vi "SetParameter.vi"(7 "Camera Parameter":T1, 8 "error in (no error)":errorcluster, 10 "Value":i32, 11 "Stream in":refnum<class "Stream.lvclass">) -> (0 "error out":errorcluster, 1 "Set Value":i32, 3 "Stream (Duplicate)":refnum<class "Stream.lvclass">)   [LabVIEW 2020, in "g_ar_toolkit.capture.lvlib" / "Stream.lvclass"]
uses:
  Stream.lvclass
  Camera Parameters.ctl
  Stream.lvclass/Stream.ctl
  g_ar_toolkit.common/g_ar_toolkit.common.lvlib
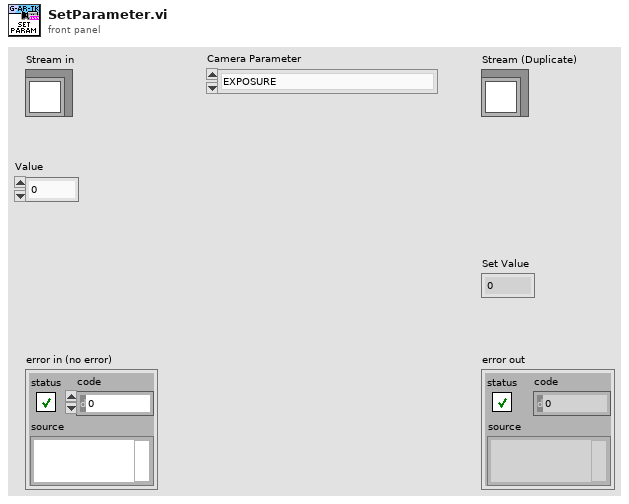
[diagram p1: front panel]
types:
  T1 = typedef "g_ar_toolkit.capture.lvlib/Stream.lvclass/Camera Parameters.ctl" = enum8{"EXPOSURE", "FOCUS", "ZOOM", "GAIN", "WHITE_BALANCE_TEMPERATURE", "BRIGHTNESS", "CONTRAST", "SATURATION", "GAMMA", "HUE", "SHARPNESS", "BACKLIGHT_COMPENSATION", "POWER_LINE_FREQUENCY"}
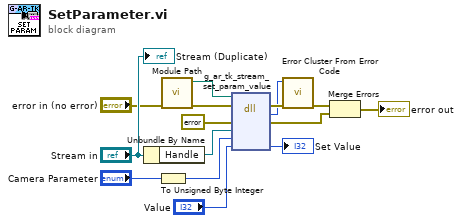
[diagram p0: block diagram]
diagram:
  n1 = Unbundle By Name("Stream in") -> ("Handle"=w11:refnum<data-value>)
  n2 = To Unsigned Byte Integer(number="Camera Parameter") -> (unsigned 8bit integer=w5:u8)
  n3 = call "Module Path.vi"("error in (no error)"="error in (no error)") -> ("error out"=w1:errorcluster, "Path"=w3:path)  [unwired: 9 in]
  n4 = dll-call lib="?" fn="g_ar_tk_stream_set_param_value" ("g_ar_toolkit.*.*:g_ar_tk_stream_capture_next")(path in=w3, error in=w1, "error_cluster"=errorcluster {"status"=FALSE, "code"=0, "source"=""} ("error constant"), "EDVR_strm"=w11, "parameter"=w5, "value"="Value") -> (error out=w10:errorcluster, "MgErr"=w9:i32, "error_cluster"=w7:errorcluster, "value"=→"Set Value":i32)  [unwired: 3 in, 1 out]
  n5 = call <vilib>:"Error Cluster From Error Code.vi"("error in (no error)"=w10, "error code (0)"=w9) -> ("error out"=w8:errorcluster)  [unwired: 7 in]
  n6 = Merge Errors(w8, w7) -> (→"error out":errorcluster)
  "Stream (Duplicate)" <- "Stream in"
